vi "Condense Histogram.vi"(11 "Histogram Graph in":T1) -> (3 "Histogram Graph out":T1)   [LabVIEW 2016]
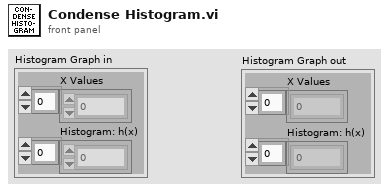
[diagram p1: front panel]
types:
  T1 = cluster{"X Values":dbl[], "Histogram: h(x)":i32[]}
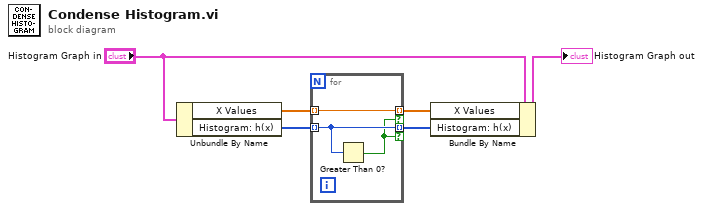
[diagram p0: block diagram]
diagram:
  n1 = Unbundle By Name("Histogram Graph in") -> ("X Values"=w5:dbl[], "Histogram: h(x)"=w4:i32[])
  n2 = for {
    tunnel: w5 -> [w9] mode=indexing
    tunnel: w4 -> [w8] mode=indexing
    tunnel: [w9] -> w3 mode=indexing if=w7
    tunnel: [w8] -> w2 mode=indexing if=w7
    n3 = Greater Than 0?(x=w8) -> (x > 0?=w7:bool)
  }
  n4 = Bundle By Name(cluster="Histogram Graph in", "X Values"=w3, "Histogram: h(x)"=w2) -> (→"Histogram Graph out":T1)
